vi "Software Update HCC Latest Data Folder.vi"(8 "error in (no error)":errorcluster, 10 "New Software Location":path, 11 "Path Build List Sub Input":path) -> (0 "error out":errorcluster, 2 "Latest Exe Files":path[](array[path]), 3 "Path Build List Sub Output":path)   [LabVIEW 2016]
panel:
  out "All Files in Dir":path[](array[path])
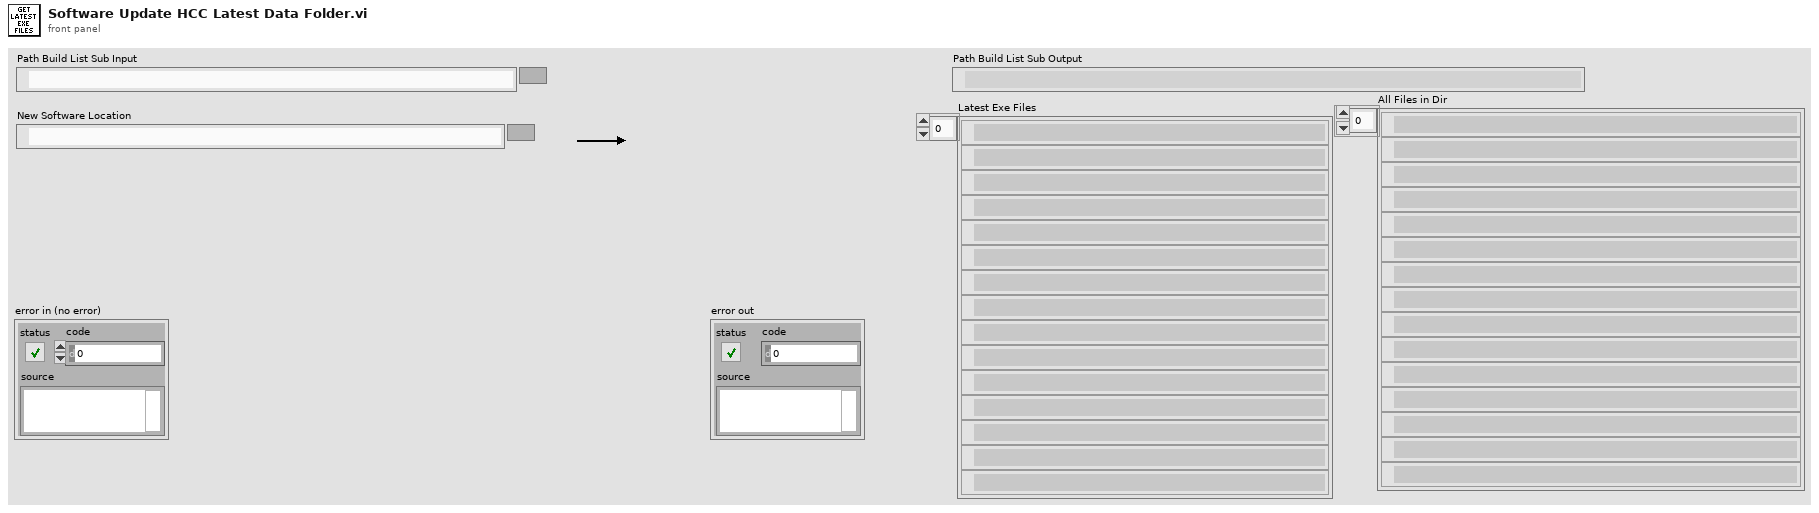
[diagram p1: front panel]
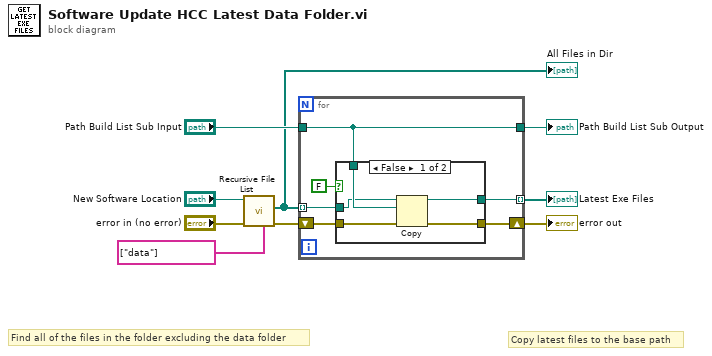
[diagram p0: block diagram]
diagram:
  # "Copy latest files to the base path"
  # "Find all of the files in the folder excluding the data folder"
  n1 = call <vilib>:"Recursive File List.vi"("Folders to Exclude"=string[] ["data"], "error in (no error)"="error in (no error)", "Folder Path"="New Software Location") -> ("error out"=w2:errorcluster, "All Files in Dir"=w3:path[])  [unwired: 4 in, 3 out]
  "All Files in Dir" <- w3
  n2 = for {
    tunnel: "Path Build List Sub Input" -> [w14]
    tunnel: w3 -> [w11] mode=indexing
    shift-right: [w13] -> w7
    shift-left: w2 -> [w15]
    tunnel: [w14] -> w5
    tunnel: [w12] -> w6 mode=indexing
    n3 = case shown="False" FALSE {
      tunnel: w15 -> [w20 w21]
      tunnel: w14 -> [w19 _]
      tunnel: [w18 w21] -> w13
      tunnel: [w17 w22] -> w12
      tunnel: w11 -> [w16 w22]
      frame False {
        n4 = Copy(8:w20, 10:w19, 11:w16) -> (0:w18:errorcluster, 3:w17:path)  [unwired: 2 in, 1 out]
      }
      frame True {
      }
    }
  }
  "error out" <- w7
  "Latest Exe Files" <- w6
  "Path Build List Sub Output" <- w5
